vi "Teleop.vi"(10 "Match Info":T1={"Autonomous Elapsed Seconds"=0.0, "TeleOp Elapsed Seconds"=0.0, "Disabled Elapsed Seconds"=0.0, "Visited Autonomous"=FALSE, "Visited TeleOp"=FALSE, "Visited Disabled"=FALSE, "Autonomous Settings"={"Autonomous Style"=enum."Independent", "VI Refnum"=refnum}}, 11 "Call Context":T2) -> ()   [LabVIEW 2017]
doc: "This VI is called for each TeleOp packet received from the DS where the robot is not disabled. It is often used to read from the joysticks and update I/O or to update setpoints for timed control loops. It should complete and return within 20 milliseconds or it may miss DS packets."
uses:
  <vilib>/Rock Robotics/WPI/DriverStation/WPI_DriverStationDerivedRobotMode.ctl
  <vilib>/Rock Robotics/WPI/DriverStation/WPI_DriverStationMatch Info.ctl
  <vilib>/Rock Robotics/WPI/Utilities/WPI_GetSetVariantRefNum.vi
  Subsystem/Drive/Drive.lvclass
  Subsystem/Intake/Intake.lvclass
  Subsystem/RobotLift/RobotLift.lvclass
  Subsystem/CubeLift/CubeLift.lvclass
panel:
  # "Intake-Collect, A - 0\nIntake-Deposit, B - 1\n\nCube Lift-Deposit, Y - 3\nCube Lift-Up, Dpad Up - 0\nCube Lift-Down, Dpad Down - 180\n\nRobot Lift - Release Ramps, X - 2\nRobot Lift - Left Up, LB - 4\nRobot Lift - Left Down, LT - Axis 2\nRobot Lift - Right Up, RB - 5\nRobot Lift - Right Down, RT - Axis 3"
  # "Right Robot Lift Up"
  # "Left Robot Lift Up"
  # "Right Robot Lift Down"
  # "Left Robot Lift Down"
  # "CubeLift-Deposit"
  # "Cube Lift Up"
  # "Intake-Deposit"
  # "RobotLift\n- Release Ramps"
  # "Cube Lift Down"
  # "Intake-Collect"
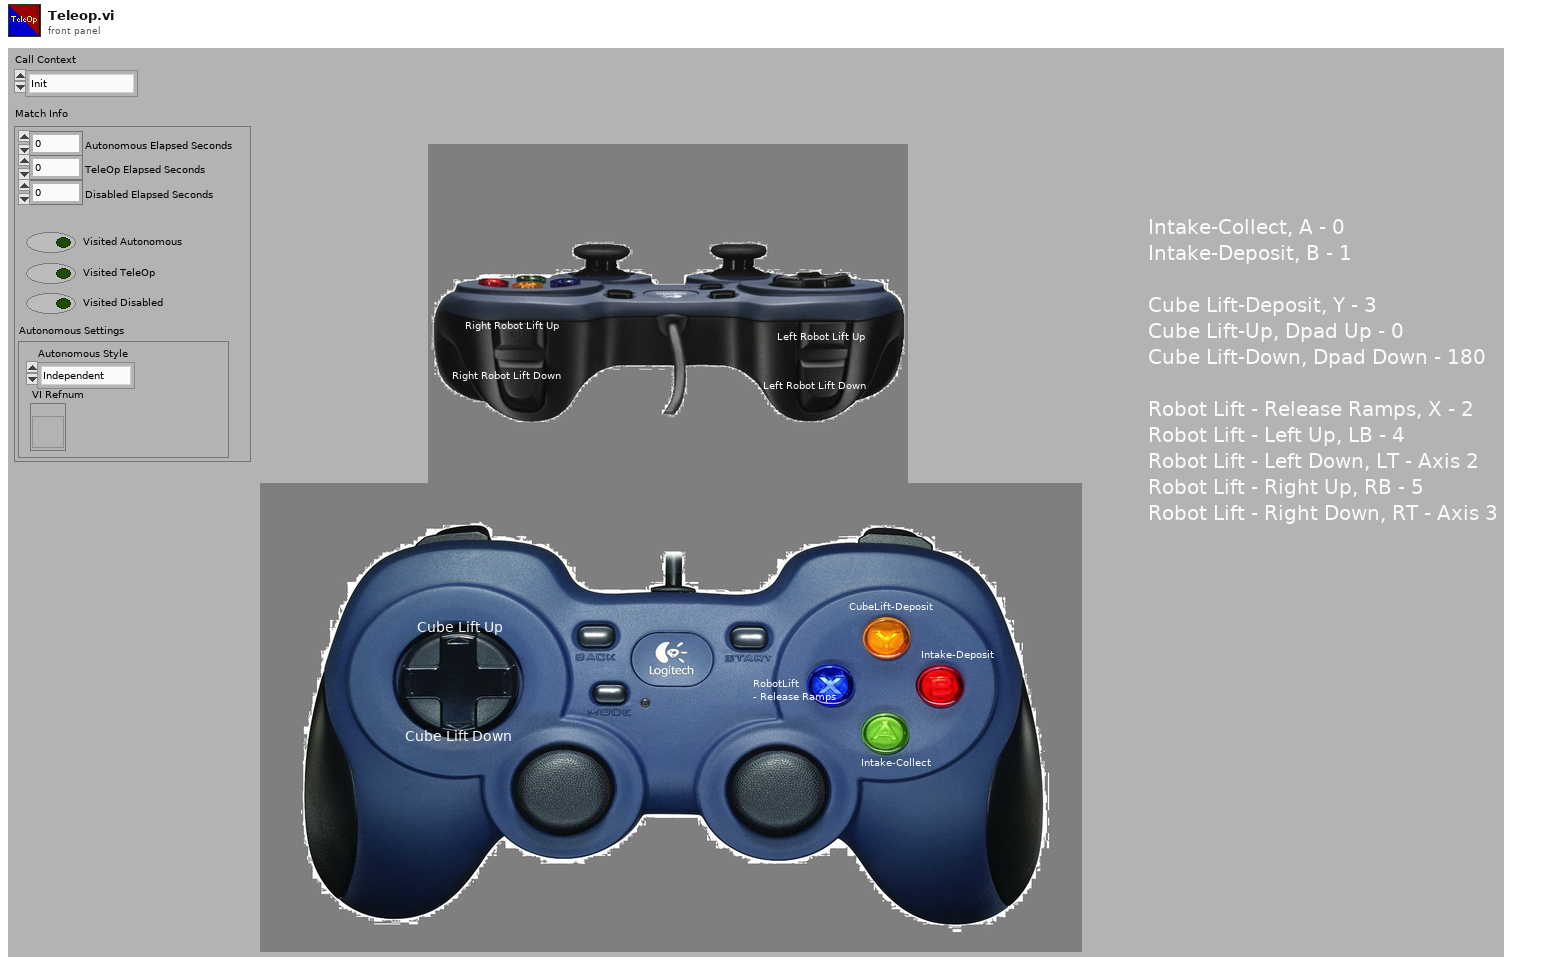
[diagram p1: front panel]
types:
  T1 = typedef "WPI_DriverStationMatch Info.ctl" = cluster{"Autonomous Elapsed Seconds":dbl, "TeleOp Elapsed Seconds":dbl, "Disabled Elapsed Seconds":dbl, "Visited Autonomous":bool, "Visited TeleOp":bool, "Visited Disabled":bool, "Autonomous Settings":cluster{"Autonomous Style":enum16{"Iterative", "Independent"}, "VI Refnum":refnum<vi>}}
  T2 = typedef "WPI_DriverStationDerivedRobotMode.ctl" = enum16{"Init", "Execute", "Stop"}
  T3 = typedef "WPI_JoystickDevRef.ctl" = cluster{"Device":T4}
  T4 = typedef "WPI_JoystickDeviceEnum.ctl" = enum16{"USB 0", "USB 1", "USB 2", "USB 3", "USB 4", "USB 5"}
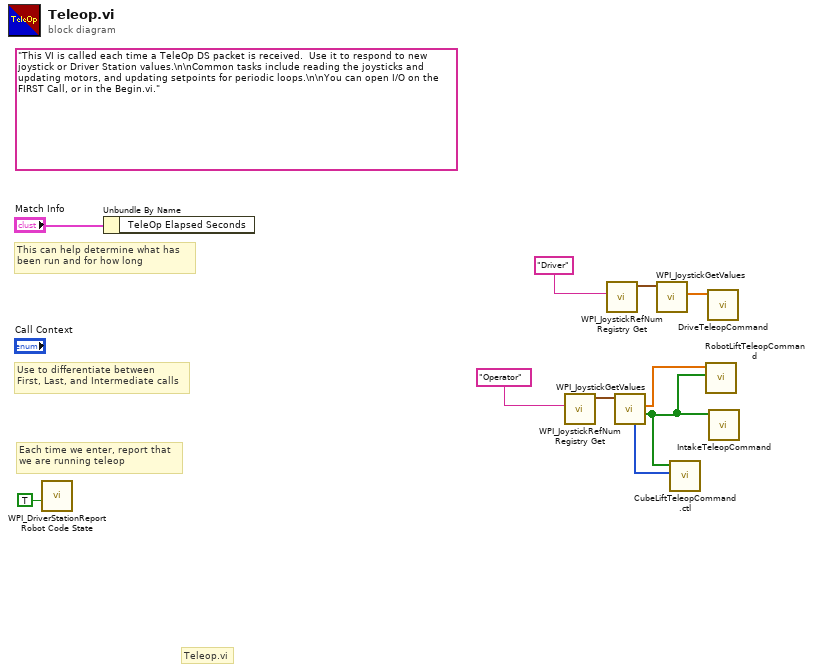
[diagram p0: block diagram]
diagram:
  (unwired) "This VI is called each time a TeleOp DS packet is received.  Use it to respond to new joystick or Driver Station values.\n\nCommon tasks include reading the joysticks and updating motors, and updating setpoints for periodic loops.\n\nYou can open I/O on the FIRST Call, or in the Begin.vi."
  # "Teleop.vi"
  # "Each time we enter, report that\nwe are running teleop"
  # "Use to differentiate between\nFirst, Last, and Intermediate calls"
  # "This can help determine what has\nbeen run and for how long"
  n1 = call <vilib>:"WPI_DriverStationReport Robot Code State.vi"("TeleOp"=TRUE ("Autonomous")) -> ()  [unwired: 10 in, 1 out]
  n2 = Unbundle By Name("Match Info") -> ()  [unwired: 1 out]
  n3 = call <vilib>:"WPI_JoystickRefNum Registry Get.vi"("refnum name"="Operator") -> ("JoystickDevRef"=w6:T3)  [unwired: 1 in, 9 out]
  n4 = call <vilib>:"WPI_JoystickRefNum Registry Get.vi"("refnum name"="Driver") -> ("JoystickDevRef"=w8:T3)  [unwired: 1 in, 9 out]
  n5 = call <vilib>:"WPI_JoystickGetValues.vi"("JoystickDevRef"=w6) -> ("Buttons"=w2:bool[], "Axes"=w3:dbl[], "POVs"=w1:i16[])  [unwired: 6 in, 2 out]
  n6 = call <vilib>:"WPI_JoystickGetValues.vi"("JoystickDevRef"=w8) -> ("Axes"=w4:dbl[])  [unwired: 6 in, 4 out]
  n7 = call "CubeLiftTeleopCommand.ctl"("POVs"=w1, "Buttons"=w2) -> ()  [unwired: 10 in]
  n8 = call "RobotLiftTeleopCommand.vi"("Buttons"=w2, "Axes"=w3) -> ()  [unwired: 10 in]
  n9 = call "DriveTeleopCommand.vi"("Axes"=w4) -> ()  [unwired: 11 in]
  n10 = call "IntakeTeleopCommand.vi"("Buttons"=w2) -> ()  [unwired: 11 in]
